vi "Frequency Counter Waveform.vi"(0 "Channel(1,2,3)":enum16{"Channel 1", "Channel 2", "Channel 3"}(ring), 7 "VISA resource name":refnum<visa-resource-name>="GPIB0::3::INSTR", 11 "error in":errorcluster) -> (2 "Symmetry":dbl format="%.6f", 3 "Frequency":dbl format="%.6f", 4 "Vmax":dbl format="%.6f", 6 "Vmin":dbl format="%.6f", 8 "RTime":dbl format="%.6f", 10 "FTime":dbl format="%.6f", 15 "error out":errorcluster)   [LabVIEW 2024]
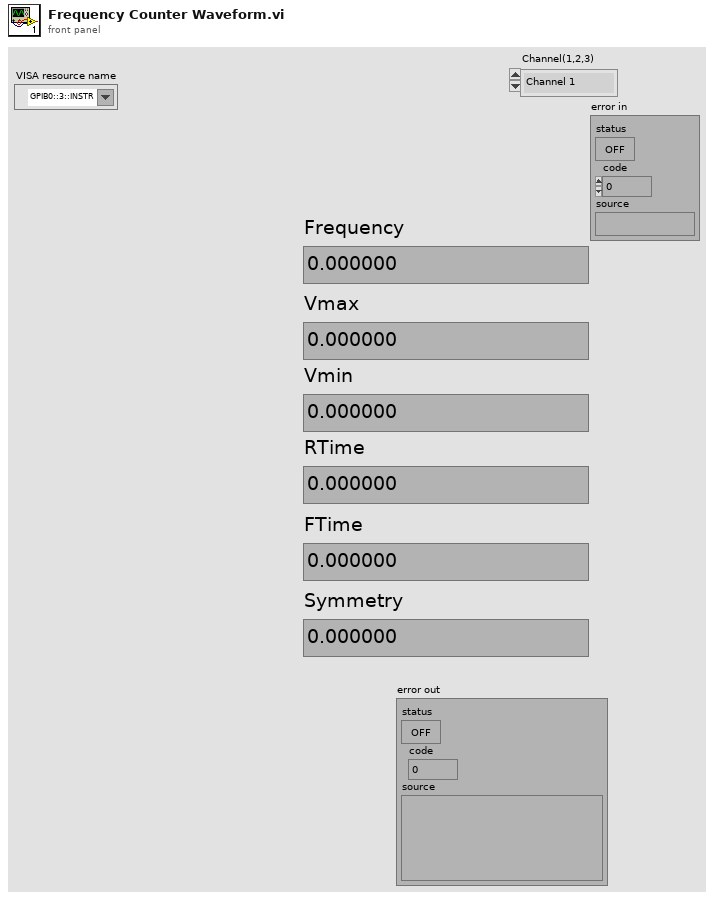
[diagram p1: front panel]
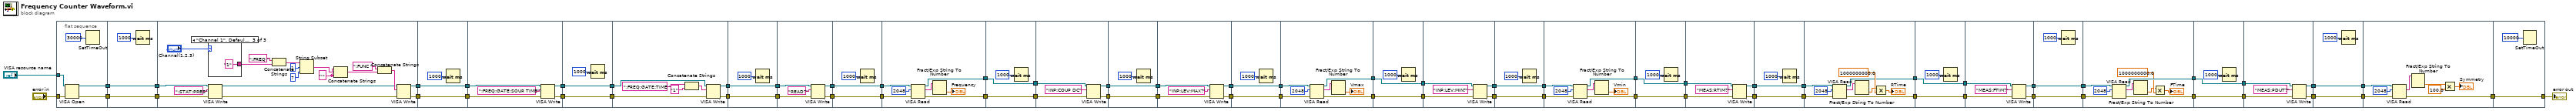
[diagram p0: block diagram]
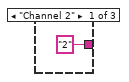
[diagram p2: hidden frame]
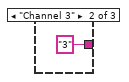
[diagram p3: hidden frame]
diagram:
  n1 = flat-sequence {
    tunnel: [w71] -> w65
    tunnel: [w72] -> w63
    tunnel: "error in" -> [w70]
    tunnel: "VISA resource name" -> [w69]
    tunnel: w65 -> [w76]
    tunnel: [w76] -> w64
    tunnel: w63 -> [w75]
    tunnel: [w75] -> w62
    tunnel: w64 -> [w81]
    tunnel: w62 -> [w80]
    tunnel: [w79] -> w61
    tunnel: [w78] -> w59
    tunnel: w61 -> [w100]
    tunnel: [w100] -> w60
    tunnel: w59 -> [w99]
    tunnel: [w99] -> w58
    tunnel: w60 -> [w104]
    tunnel: w58 -> [w103]
    tunnel: [w102] -> w57
    tunnel: [w101] -> w55
    tunnel: w57 -> [w108]
    tunnel: [w108] -> w56
    tunnel: w55 -> [w107]
    tunnel: [w107] -> w54
    tunnel: w56 -> [w112]
    tunnel: w54 -> [w111]
    tunnel: [w110] -> w53
    tunnel: [w109] -> w51
    tunnel: w53 -> [w118]
    tunnel: [w118] -> w52
    tunnel: w51 -> [w117]
    tunnel: [w117] -> w50
    tunnel: w52 -> [w122]
    tunnel: w50 -> [w121]
    tunnel: [w120] -> w49
    tunnel: [w119] -> w47
    tunnel: w49 -> [w126]
    tunnel: [w126] -> w48
    tunnel: w47 -> [w125]
    tunnel: [w125] -> w46
    tunnel: w48 -> [w131]
    tunnel: w46 -> [w130]
    tunnel: [w128] -> w45
    tunnel: [w127] -> w43
    tunnel: w45 -> [w136]
    tunnel: [w136] -> w44
    tunnel: w43 -> [w135]
    tunnel: [w135] -> w42
    tunnel: w44 -> [w140]
    tunnel: w42 -> [w139]
    tunnel: [w138] -> w41
    tunnel: [w137] -> w39
    tunnel: w41 -> [w144]
    tunnel: [w144] -> w40
    tunnel: w39 -> [w143]
    tunnel: [w143] -> w38
    tunnel: w40 -> [w149]
    tunnel: w38 -> [w148]
    tunnel: [w147] -> w37
    tunnel: [w146] -> w35
    tunnel: w37 -> [w152]
    tunnel: [w152] -> w36
    tunnel: w35 -> [w151]
    tunnel: [w151] -> w34
    tunnel: w36 -> [w157]
    tunnel: w34 -> [w156]
    tunnel: [w155] -> w33
    tunnel: [w154] -> w31
    tunnel: w33 -> [w162]
    tunnel: [w162] -> w32
    tunnel: w31 -> [w161]
    tunnel: [w161] -> w30
    tunnel: w32 -> [w165]
    tunnel: w30 -> [w167]
    tunnel: [w164] -> w29
    tunnel: [w163] -> w27
    tunnel: w29 -> [w170]
    tunnel: [w170] -> w28
    tunnel: w27 -> [w169]
    tunnel: [w169] -> w26
    tunnel: w28 -> [w175]
    tunnel: w26 -> [w174]
    tunnel: [w173] -> w25
    tunnel: [w172] -> w23
    tunnel: w25 -> [w180]
    tunnel: [w180] -> w24
    tunnel: w23 -> [w179]
    tunnel: [w179] -> w22
    tunnel: w24 -> [w183]
    tunnel: w22 -> [w185]
    tunnel: [w182] -> w21
    tunnel: [w181] -> w19
    tunnel: w21 -> [w188]
    tunnel: [w188] -> w20
    tunnel: w19 -> [w187]
    tunnel: [w187] -> w18
    tunnel: w20 -> [w194]
    tunnel: w18 -> [w193]
    tunnel: [w191] -> w5
    tunnel: [w190] -> w3
    tunnel: w5 -> [w200]
    tunnel: [w200] -> w4
    tunnel: w3 -> [w199]
    tunnel: [w199] -> w2
    tunnel: w4 -> [w203]
    tunnel: w2 -> [w205]
    tunnel: [w202] -> w9
    tunnel: [w201] -> w7
    tunnel: w9 -> [w208]
    tunnel: [w208] -> w8
    tunnel: w7 -> [w207]
    tunnel: [w207] -> w6
    tunnel: w8 -> [w216]
    tunnel: w6 -> [w215]
    tunnel: [w214] -> w13
    tunnel: [w213] -> w11
    tunnel: w13 -> [w220]
    tunnel: [w220] -> w12
    tunnel: w11 -> [w219]
    tunnel: [w219] -> w10
    tunnel: w12 -> [w225]
    tunnel: w10 -> [w223]
    tunnel: [w222] -> w17
    tunnel: [w221] -> w15
    tunnel: w17 -> [w228]
    tunnel: [w228] -> w16
    tunnel: w15 -> [w227]
    tunnel: [w227] -> w14
    tunnel: w16 -> [w233]
    tunnel: w14 -> [w232]
    tunnel: [w230] -> w67
    tunnel: w67 -> [w237]
    tunnel: [w237] -> w66
    frame #0 {
      n2 = VISA Open(error in (no error)=w70, VISA resource name=w69) -> (VISA resource name=w71:refnum<visa-resource-name>, error out=w72:errorcluster)  [unwired: 3 in]
      n3 = SetTimeOut(1:30000) -> ()  [unwired: 1 out]
    }
    frame #1 {
      n4 = Wait (ms)(milliseconds to wait=u32 1000) -> ()  [unwired: 1 out]
    }
    frame #2 {
      w85 = "'"
      n5 = case shown="\"Channel 1\", Default" "Channel(1,2,3)" {
        tunnel: ["2" "3" "1"] -> w91
        frame "Channel 2" {
        }
        frame "Channel 3" {
        }
        frame "Channel 1", Default {
        }
      }
      n6 = VISA Write(VISA resource name=w81, write buffer=":STAT:PRES" ("data string"), error in (no error)=w80) -> (VISA resource name out=w83:refnum<visa-resource-name>, error out=w82:errorcluster)  [unwired: 1 out]
      n7 = Concatenate Strings(":FREQ ", w91) -> (w89:string)
      n8 = String Subset(string=w89, offset (0)=1, length (rest)=7 ("length (rest)")) -> (substring=w86:string)
      n9 = Concatenate Strings(w85, w86, w85) -> (w84:string)
      n10 = Concatenate Strings(":FUNC " ("data string"), w84) -> (w92:string)
      n11 = VISA Write(VISA resource name=w83, write buffer=w92, error in (no error)=w82) -> (VISA resource name out=w79:refnum<visa-resource-name>, error out=w78:errorcluster)  [unwired: 1 out]
    }
    frame #3 {
      n12 = Wait (ms)(milliseconds to wait=u32 1000) -> ()  [unwired: 1 out]
    }
    frame #4 {
      n13 = VISA Write(VISA resource name=w104, write buffer=":FREQ:GATE:SOUR TIME" ("data string"), error in (no error)=w103) -> (VISA resource name out=w102:refnum<visa-resource-name>, error out=w101:errorcluster)  [unwired: 1 out]
    }
    frame #5 {
      n14 = Wait (ms)(milliseconds to wait=u32 1000) -> ()  [unwired: 1 out]
    }
    frame #6 {
      n15 = Concatenate Strings(":FREQ:GATE:TIME " ("data string"), "1" ("string")) -> (w113:string)
      n16 = VISA Write(VISA resource name=w112, write buffer=w113, error in (no error)=w111) -> (VISA resource name out=w110:refnum<visa-resource-name>, error out=w109:errorcluster)  [unwired: 1 out]
    }
    frame #7 {
      n17 = Wait (ms)(milliseconds to wait=u32 1000) -> ()  [unwired: 1 out]
    }
    frame #8 {
      n18 = VISA Write(VISA resource name=w122, write buffer="READ?" ("data string"), error in (no error)=w121) -> (VISA resource name out=w120:refnum<visa-resource-name>, error out=w119:errorcluster)  [unwired: 1 out]
    }
    frame #9 {
      n19 = Wait (ms)(milliseconds to wait=u32 1000) -> ()  [unwired: 1 out]
    }
    frame #10 {
      n20 = VISA Read(VISA resource name=w131, byte count=u32 2048, error in (no error)=w130) -> (VISA resource name out=w128:refnum<visa-resource-name>, read buffer=w133:string, error out=w127:errorcluster)  [unwired: 1 out]
      n21 = Fract/Exp String To Number(string=w133) -> (number=→"Frequency":dbl)  [unwired: 3 in, 1 out]
    }
    frame #11 {
      n22 = Wait (ms)(milliseconds to wait=u32 1000) -> ()  [unwired: 1 out]
    }
    frame #12 {
      n23 = VISA Write(VISA resource name=w140, write buffer="INP:COUP DC" ("data string"), error in (no error)=w139) -> (VISA resource name out=w138:refnum<visa-resource-name>, error out=w137:errorcluster)  [unwired: 1 out]
    }
    frame #13 {
      n24 = Wait (ms)(milliseconds to wait=u32 1000) -> ()  [unwired: 1 out]
    }
    frame #14 {
      n25 = VISA Write(VISA resource name=w149, write buffer="INP:LEV:MAX?" ("data string"), error in (no error)=w148) -> (VISA resource name out=w147:refnum<visa-resource-name>, error out=w146:errorcluster)  [unwired: 1 out]
    }
    frame #15 {
      n26 = Wait (ms)(milliseconds to wait=u32 1000) -> ()  [unwired: 1 out]
    }
    frame #16 {
      n27 = VISA Read(VISA resource name=w157, byte count=u32 2048, error in (no error)=w156) -> (VISA resource name out=w155:refnum<visa-resource-name>, read buffer=w158:string, error out=w154:errorcluster)  [unwired: 1 out]
      n28 = Fract/Exp String To Number(string=w158) -> (number=→"Vmax":dbl)  [unwired: 3 in, 1 out]
    }
    frame #17 {
      n29 = Wait (ms)(milliseconds to wait=u32 1000) -> ()  [unwired: 1 out]
    }
    frame #18 {
      n30 = VISA Write(VISA resource name=w165, write buffer="INP:LEV:MIN?" ("data string"), error in (no error)=w167) -> (VISA resource name out=w163:refnum<visa-resource-name>, error out=w164:errorcluster)  [unwired: 1 out]
    }
    frame #19 {
      n31 = Wait (ms)(milliseconds to wait=u32 1000) -> ()  [unwired: 1 out]
    }
    frame #20 {
      n32 = VISA Read(VISA resource name=w174, byte count=u32 2048, error in (no error)=w175) -> (VISA resource name out=w173:refnum<visa-resource-name>, read buffer=w176:string, error out=w172:errorcluster)  [unwired: 1 out]
      n33 = Fract/Exp String To Number(string=w176) -> (number=→"Vmin":dbl)  [unwired: 3 in, 1 out]
    }
    frame #21 {
      n34 = Wait (ms)(milliseconds to wait=u32 1000) -> ()  [unwired: 1 out]
    }
    frame #22 {
      n35 = VISA Write(VISA resource name=w183, write buffer="MEAS:RTIM?" ("data string"), error in (no error)=w185) -> (VISA resource name out=w181:refnum<visa-resource-name>, error out=w182:errorcluster)  [unwired: 1 out]
    }
    frame #23 {
      n36 = Wait (ms)(milliseconds to wait=u32 1000) -> ()  [unwired: 1 out]
    }
    frame #24 {
      n37 = VISA Read(VISA resource name=w193, byte count=u32 2048, error in (no error)=w194) -> (VISA resource name out=w191:refnum<visa-resource-name>, read buffer=w196:string, error out=w190:errorcluster)  [unwired: 1 out]
      n38 = Fract/Exp String To Number(string=w196) -> (number=w197:dbl)  [unwired: 3 in, 1 out]
      n39 = Multiply(x=w197, y=1000000000.0) -> (x*y=→"RTime":dbl)
    }
    frame #25 {
      n40 = Wait (ms)(milliseconds to wait=u32 1000) -> ()  [unwired: 1 out]
    }
    frame #26 {
      n41 = VISA Write(VISA resource name=w203, write buffer="MEAS:FTIM?" ("data string"), error in (no error)=w205) -> (VISA resource name out=w201:refnum<visa-resource-name>, error out=w202:errorcluster)  [unwired: 1 out]
    }
    frame #27 {
      n42 = Wait (ms)(milliseconds to wait=u32 1000) -> ()  [unwired: 1 out]
    }
    frame #28 {
      n43 = VISA Read(VISA resource name=w215, byte count=u32 2048, error in (no error)=w216) -> (VISA resource name out=w213:refnum<visa-resource-name>, read buffer=w217:string, error out=w214:errorcluster)  [unwired: 1 out]
      n44 = Fract/Exp String To Number(string=w217) -> (number=w210:dbl)  [unwired: 3 in, 1 out]
      n45 = Multiply(x=w210, y=1000000000.0) -> (x*y=→"FTime":dbl)
    }
    frame #29 {
      n46 = Wait (ms)(milliseconds to wait=u32 1000) -> ()  [unwired: 1 out]
    }
    frame #30 {
      n47 = VISA Write(VISA resource name=w223, write buffer="MEAS:PDUT?" ("data string"), error in (no error)=w225) -> (VISA resource name out=w221:refnum<visa-resource-name>, error out=w222:errorcluster)  [unwired: 1 out]
    }
    frame #31 {
      n48 = Wait (ms)(milliseconds to wait=u32 1000) -> ()  [unwired: 1 out]
    }
    frame #32 {
      n49 = VISA Read(VISA resource name=w232, byte count=u32 2048, error in (no error)=w233) -> (read buffer=w235:string, error out=w230:errorcluster)  [unwired: 2 out]
      n50 = Fract/Exp String To Number(string=w235) -> (number=w236:dbl)  [unwired: 3 in, 1 out]
      n51 = Multiply(x=w236, y=100.0) -> (x*y=→"Symmetry":dbl)
    }
    frame #33 {
      n52 = SetTimeOut(1:10000 ("new timeout (10000)")) -> ()  [unwired: 1 out]
    }
  }
  "error out" <- w66
